vi "Robot Global Data.vi"() -> ()   [LabVIEW 2013]
doc: "This global VI can contain as many global variables as you need. Place a control on the panel, give it a good name. To read or write to it from a VI, drag the icon to the diagram of that VI. You can also drag from the project. Click on the node to change which global you access. You shouldn't have multiple locations writing to a global or it will cause a race-condition."
uses:
  <vilib>/Rock Robotics/WPI/Camera/WPI_CameraImageSize.ctl
  <vilib>/Rock Robotics/WPI/DriverStation/WPI_DriverStationRobotMode2.ctl
  <vilib>/Rock Robotics/WPI/Joystick/WPI_JoystickButtonState.ctl
  <vilib>/Rock Robotics/WPI/Solenoid/WPI_SolenoidValue.ctl
panel:
  in  "Auto Settings":T1
  in  "Shot duration":dbl
  out "Firing":bool
  in  "Fake LS":bool
  in  "Output Values":T3={"Drive Output Values"=[], "Shooter Solenoid"=enum."Off", "Pickup Solenoid"=enum."On"}
  in  "Sensor input":T4
  in  "Robot Code Version":string
  in  "Mapped Input":T5
  in  "Joystick 2 Input":T7
  in  "Joystick 1 Input":T7
  in  "Joystick Config":T8(ring)
  in  "Robot Config":T9(ring)
  in  "Robot Mode":T10
  in  "LED toggle rate (ms)":u32=20
  in  "image size":T11=enum."320x240"
  in  "Enable Vision":bool
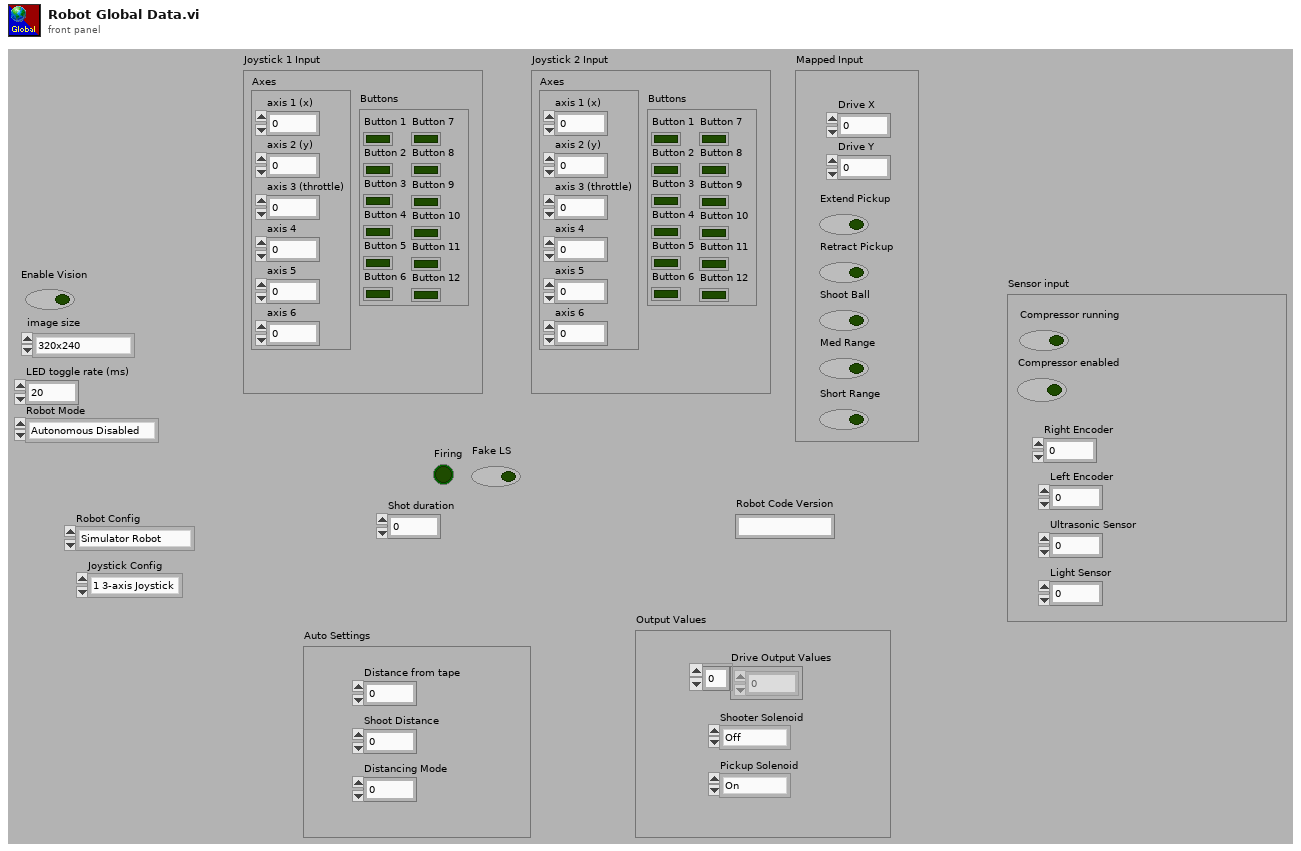
[diagram p1: front panel]
types:
  T1 = cluster{"Distance from tape":dbl, "Shoot Distance":dbl, "Distancing Mode":dbl}
  T2 = typedef "WPI_SolenoidValue.ctl" = enum16{"Off", "On", "Forward", "Reverse"}
  T3 = cluster{"Drive Output Values":dbl[], "Shooter Solenoid":T2, "Pickup Solenoid":T2}
  T4 = cluster{"Compressor running":bool, "Compressor enabled":bool, "Right Encoder":dbl, "Left Encoder":dbl, "Ultrasonic Sensor":dbl, "Light Sensor":dbl}
  T5 = cluster{"Drive Y":dbl, "Drive X":dbl, "Extend Pickup":bool, "Retract Pickup":bool, "Shoot Ball":bool, "Med Range":bool, "Short Range":bool}
  T6 = typedef "WPI_JoystickButtonState.ctl" = cluster{"Button 1":bool, "Button 2":bool, "Button 3":bool, "Button 4":bool, "Button 5":bool, "Button 6":bool, "Button 7":bool, "Button 8":bool, "Button 9":bool, "Button 10":bool, "Button 11":bool, "Button 12":bool}
  T7 = cluster{"Axes":cluster{"axis 1 (x)":dbl, "axis 2 (y)":dbl, "axis 3 (throttle)":dbl, "axis 4":dbl, "axis 5":dbl, "axis 6":dbl}, "Buttons":T6}
  T8 = enum16{"1 3-axis Joystick", "2 2-axis Joysticks"}
  T9 = enum16{"Simulator Robot", "Alpinista", "2014 Robot"}
  T10 = typedef "WPI_DriverStationRobotMode2.ctl" = enum16{"Autonomous Disabled", "Autonomous Enabled", "Teleop Disabled", "Teleop Enabled", "Timeout", "Finish", "Test Disabled", "Test Enabled"}
  T11 = typedef "WPI_CameraImageSize.ctl" = enum16{"640x480", "320x240", "160x120"}
diagram:
